vi "set trig out before integration.vi"(8 "error in (no error)":errorcluster, 11 "LineCCD in":refnum<class "LineCCD.lvclass">) -> (0 "error out":errorcluster, 3 "LineCCD out":refnum<class "LineCCD.lvclass">)   [LabVIEW 2012, in "LineCCD.lvclass"]
uses:
  LineCCD.lvclass
  LineCCD.lvclass/LineCCD.ctl
  <instrlib>/ALPHALAS CCD S Series/ALPHALAS CCD S Series.lvlib
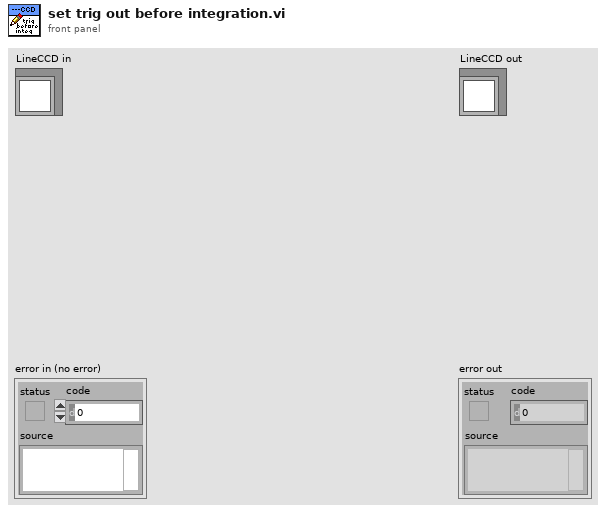
[diagram p1: front panel]
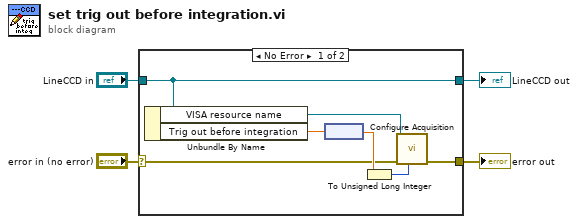
[diagram p0: block diagram]
diagram:
  n1 = case shown="No Error" "error in (no error)" {
    selector: "error in (no error)" -> [w7 w13]
    tunnel: [w6 w13] -> w3
    tunnel: [w8 w12] -> w1
    tunnel: "LineCCD in" -> [w8 w12]
    frame No Error {
      n2 = Unbundle By Name(w8) -> ("VISA resource name"=w9:refnum<visa-resource-name>, "Trig out before integration"=w10:dbl[unit])
      n3 = node(w10) -> (w11:dbl)
      n4 = To Unsigned Long Integer(number=w11) -> (unsigned 32bit integer=w5:u32)
      n5 = call <instrlib>:"Configure Acquisition.vi"("Trig Out Before Integration (0 µs)"=w5, "error in (no error)"=w7, "VISA resource name"=w9) -> ("error out"=w6:errorcluster)  [unwired: 7 in, 1 out]
    }
    frame Error {
    }
  }
  "error out" <- w3
  "LineCCD out" <- w1
